vi "Untitled 1.vi"() -> ()   [LabVIEW 2016]
uses:
  PC/llb/granula_llb.lvlib
panel:
  out "текущее время":string
  out "ВЫХОД 2":bool
  in  "x140":i32
  in  "x200":i32
  in  "x240":i32
  in  "y60":i32
  in  "y120":i32
  in  "x100":i32
  in  "x300":i32
  in  "x340":i32
  in  "x400":i32
  in  "Запись отчета":bool
  in  "V7045_I_ist":dbl
  out "U_ist":string caption="Voltage (V)"
  in  "V7045_U_ist":dbl
  out "Диаметр заг.":string caption="Diameter (mm)"
  in  "out":dbl
  out "Boolean":bool
  in  "PV_зазор":dbl
  in  "задание тока А":string caption="Задание, А"
  in  "Скорость ПП 2":string caption="Plasmatron speed (mm/min)"
  in  "Скорость ПП":string caption="Longitudial speed (mm/min)"
  out "Полож плазм кон":bool caption="Конец"
  out "Полож плазм сер":bool caption="Пром."
  out "Полож заг сер":bool
  out "Полож заг нач":bool caption="НАЧАЛО"
  out "Полож заг кон":bool
  out "Полож плазм  нач":bool caption="Начало"
  out "PE2 5":string caption="Вакуум в камере\nPT2 (torr)"
  out "PE1 4":string caption="Вакуум в камере\nPT2 (torr)"
  out "PE3 5":string caption="Вакуум в камере\nPT2 (torr)"
  in  "PE1 3":dbl
  in  "PE2 4":dbl
  in  "PE3 4":dbl
  out "ИНдикатор положения полки":string
  out "P plasmatron (bar)":string
  out "P camera (bar)":string
  out "Air 2":bool
  out "Water-1 2":bool
  out "Water-2 2":bool
  out "Air 4":bool
  out "PT 8":string caption="Вакуум в камере\nPT2 (torr)"
  out "PT 7":string caption="Вакуум в камере\nPT2 (torr)"
  out "PT 6":string caption="Вакуум в камере\nPT2 (torr)"
  in  "PT1 2":dbl
  in  "PT2 2":dbl
  in  "PT3 3":dbl
  out "PT 5":string caption="Вакуум в камере\nPT2 (torr)"
  in  "PT3 2":dbl
  out "X100":bool[](array[boolean])
  out "X140":bool[](array[boolean])
  out "X200":bool[](array[boolean])
  out "X240":bool[](array[boolean])
  out "X300":bool[](array[boolean])
  out "X340":bool[](array[boolean])
  out "X400":bool[](array[boolean])
  out "Y60":bool[](array[boolean])
  out "Y120":bool[](array[boolean])
  in  "Ошибка":i16
  in  "Т1":dbl
  in  "Т2":dbl
  in  "Т3":dbl
  in  "Т4":dbl
  in  "Т5":dbl
  out "V вращ. бараб":string caption="Rotation frequency (r/min)"
  in  "V барабаны":dbl
  out "V заготовки":string
  out "V задания":string caption="Rotation speed (r/min)"
  in  "V барабаны задание":dbl
  in  "Скорость пп":i16
  in  "ЗАДАНИЕ ТОКА":i16
  in  "откачка стоп индик 3":bool
  out "ПОДШ. 1.1":string caption="T1 (C°)"
  out "ПОДШ. 1.2":string caption="T2 (C°)"
  out "ПОДШ. 2.1":string caption="T3 (C°)"
  out "ПОДШ. 2.2":string caption="T4 (C°)"
  out "ТЕМП РОЛИК":string caption="T roller (C°)"
  out "ТЕМП КАМЕРА":string caption="T gas (C°)"
  in  "Т6":dbl
  in  "Скорость пп 2":i16
  out "V барабаны 2":dbl
  out "voto plasmatron":string caption="MOTO\nPLASMATRON"
  in  "M_PLasmatron":dbl
  out "VOLTAGE":dbl(graph)
  out "CURRENT":dbl(graph)
  out "LONGITUDINAL FEED":dbl(graph)
  out "PV":dbl(graph)
  out "PULLEYS":dbl(graph)
  out "max Speed":string caption="Max speed (r/min)"
  in  "Position (mm)":dbl(slide) scale=0.0..820.0
  out "String":string
  out "ролик_прижат":bool caption="Down"
  out "ролик_отжат":bool caption="Up"
  out "УГ_открыт":bool caption="Open"
  out "УГ_закрыт":bool caption="Close"
  in  "Выход":bool
  in  "Tab Control":enum32{"VACUUM"}(tab)
  out "PT3":u16(ring)
  out "PT 3":string caption="Вакуум в камере\nPT2 (torr)"
  out "PA":string
  out "PD1":u16(ring)
  out "VP8":u16(ring)
  out "PA1":string
  out "PD2":u16(ring)
  in  "forvacuum":bool
  in  "forvakuum led":bool
  in  "Slide":dbl(slide) scale=0.0..99.0
  out "NL 2":u16(ring)
  out "VP9":u16(ring)
  in  "ND HEAT BUT":bool
  in  "ND HEAT LED":bool
  in  "откачка стоп 2":bool
  in  "откачка стоп индик 2":bool
  out "Water-2":bool
  out "Water-1":bool
  out "Air":bool
  in  "откачка стоп":bool
  in  "откачка стоп индик":bool
  out "EV1":u16(ring)
  out "EV2":u16(ring)
  out "EV3.3":u16(ring)
  out "EV3.2":u16(ring)
  out "PE2":u16(ring)
  out "PE2":string caption="Вакуум в камере\nPT2 (torr)"
  out "CO1":u16(ring)
  out "CO2":u16(ring)
  out "EV3.1":u16(ring)
  out "CO3":u16(ring)
  out "P1":u16(ring)
  out "PE1":u16(ring)
  out "PE1":string caption="Вакуум в камере\nPT2 (torr)"
  out "PE3":u16(ring)
  out "PE3":string caption="Вакуум в камере\nPT2 (torr)"
  out "VP1":u16(ring)
  out "VP2":u16(ring)
  out "PT2":u16(ring)
  out "PT 2":string caption="Вакуум в камере\nPT2 (torr)"
  out "VP3":u16(ring)
  out "VP5":u16(ring)
  out "PT1":u16(ring)
  out "PT 1":string caption="Вакуум в камере\nPT2 (torr)"
  out "NZ":u16(ring)
  out "NB":u16(ring)
  out "NL":u16(ring)
  out "VP7":u16(ring)
  in  "mac 4":bool
  in  "напустить аргон":bool
  in  "откачать рабочий вакуум":bool
  in  "mac 2":bool
  # "VF1"
  # "Ar,He"
  # "PC1"
  # "PC2"
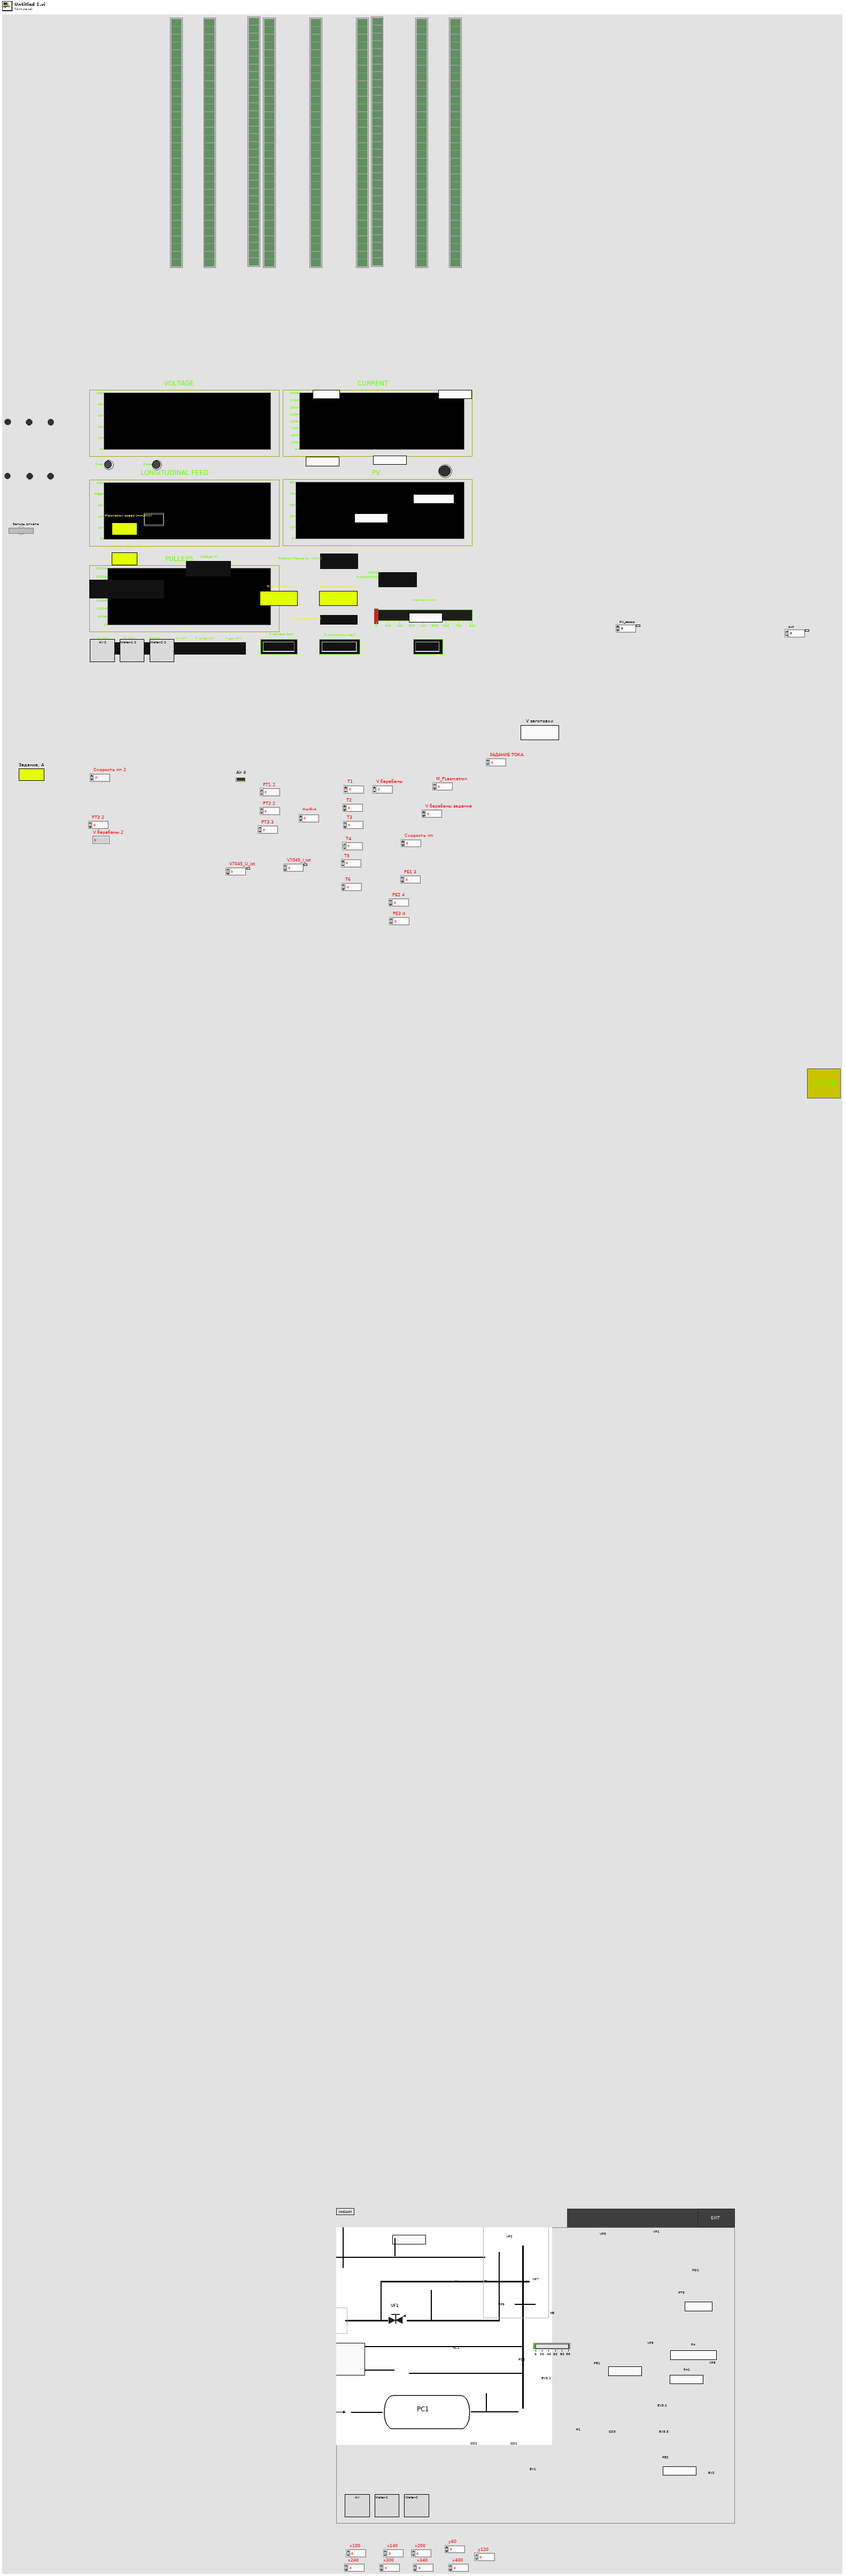
[diagram p1: front panel]
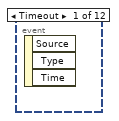
[diagram p2: hidden frame]
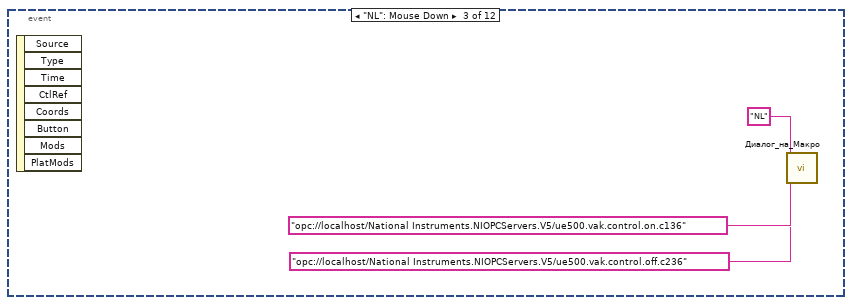
[diagram p3: hidden frame]
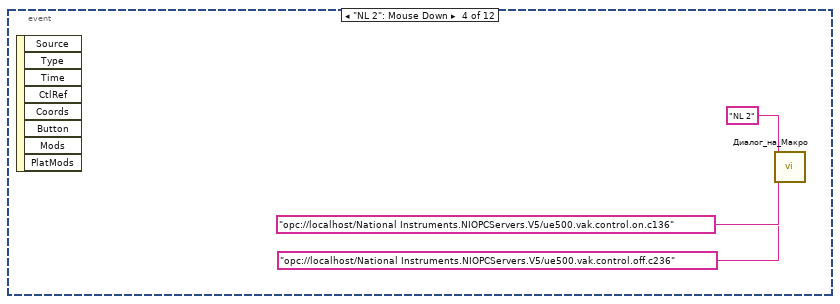
[diagram p4: hidden frame]
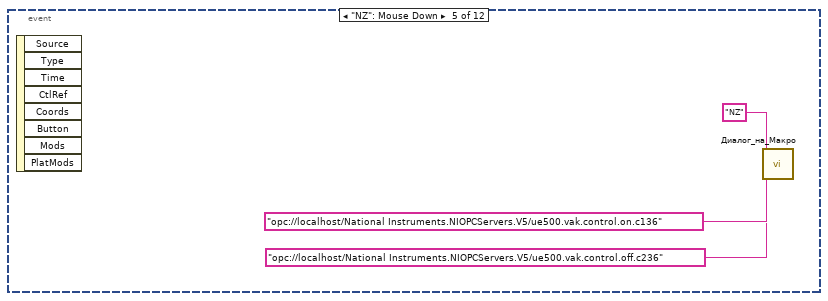
[diagram p5: hidden frame]
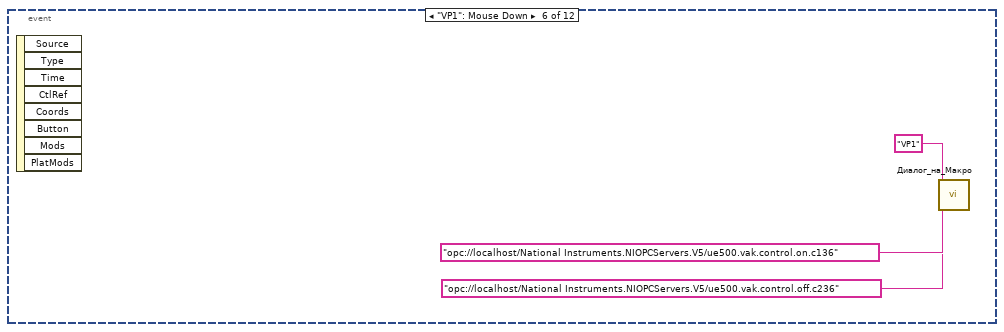
[diagram p6: hidden frame]
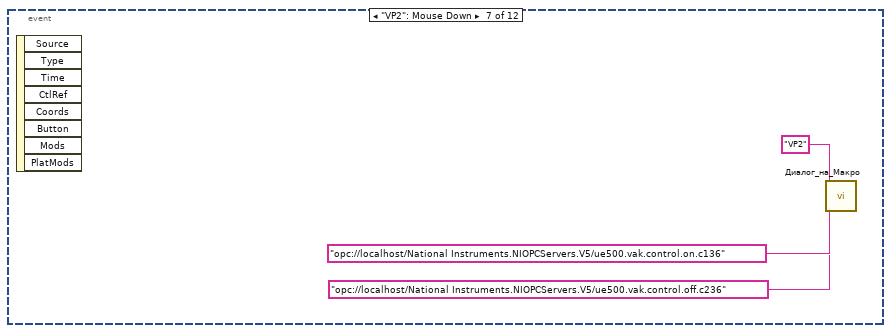
[diagram p7: hidden frame]
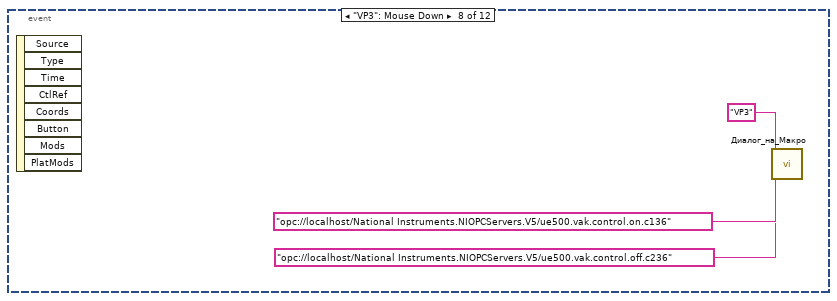
[diagram p8: hidden frame]
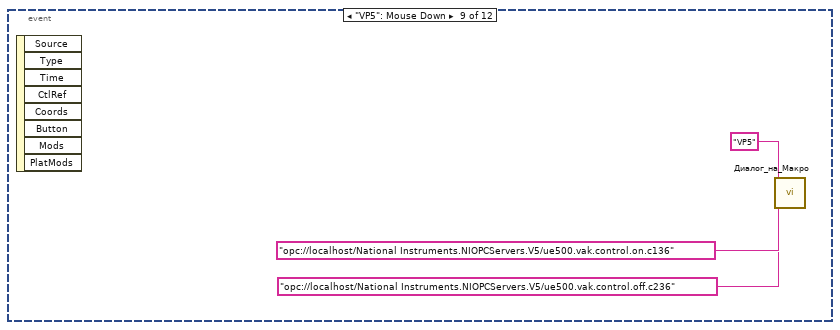
[diagram p9: hidden frame]
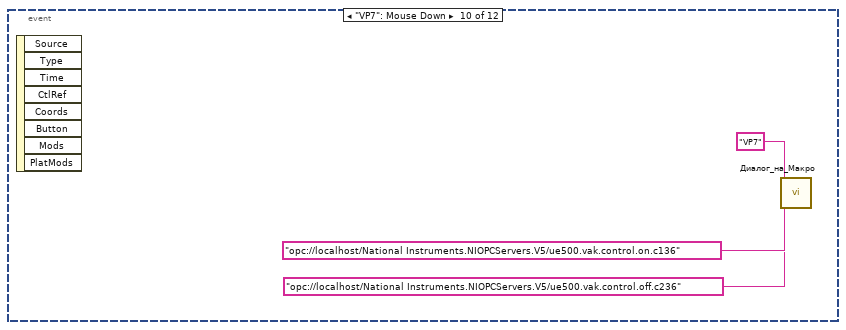
[diagram p10: hidden frame]
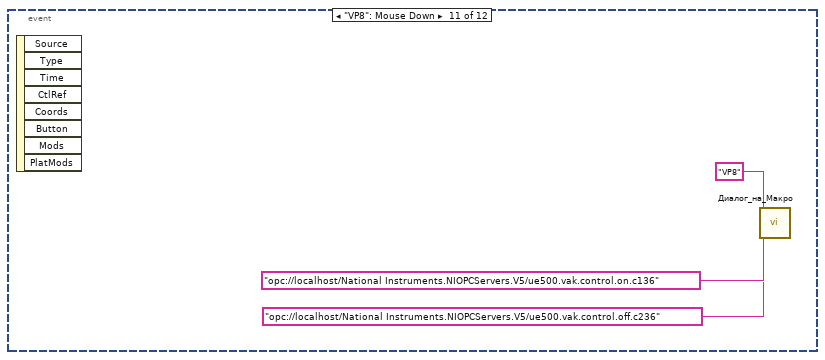
[diagram p11: hidden frame]
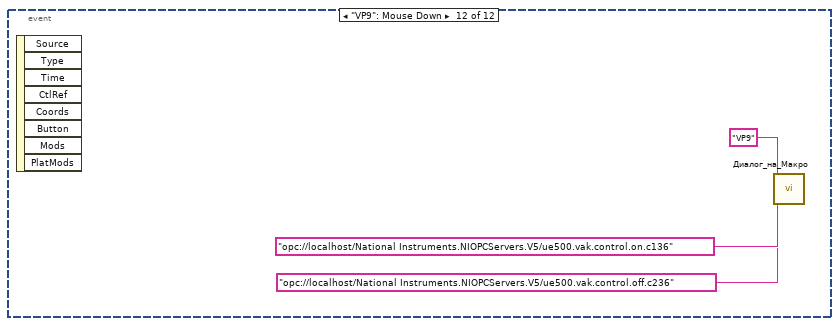
[diagram p12: hidden frame]
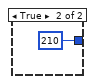
[diagram p13: hidden frame]
diagram:
  n1 = flat-sequence {
    frame #0 {
      n2 = while {
        stop <- FALSE stop-if-true
        w110 = i16 1 ("precision (6)")
        # "Вакуумная"
        n3 = local read "Y120"() -> (w228:bool[])
        n4 = local read "X200"() -> (w290:bool[])
        n5 = local read "X240"() -> (w274:bool[])
        n6 = local read "X100"() -> (w126:bool[])
        n7 = local read "X300"() -> (w249:bool[])
        n8 = local read "X340"() -> (w235:bool[])
        n9 = local read "X140"() -> (w309:bool[])
        n10 = local read "X400"() -> (w176:bool[])
        n11 = local read "Y60"() -> (w229:bool[])
        n12 = local read "out"() -> (→"LONGITUDINAL FEED":dbl)
        n13 = Get Date/Time In Seconds() -> (seconds since 1Jan1904=w183:timestamp)
        n14 = Wait Until Next ms Multiple(millisecond multiple=u32 500) -> ()  [unwired: 1 out]
        n15 = local read "V7045_U_ist"() -> (→"VOLTAGE":dbl)
        n16 = local read "V7045_I_ist"() -> (→"CURRENT":dbl)
        n17 = local read "PV_зазор"() -> (→"PV":dbl)
        n18 = local read "X140"() -> (w153:bool[])
        n19 = call "Метакон.vi"("Vak_in"="PT2 2") -> ("Vak_out_txt"=→"PT 7":string)  [unwired: 9 in, 1 out]
        n20 = call "Метакон.vi"("Vak_in"="PT3 3") -> ("Vak_out_txt"=→"PT 6":string)  [unwired: 9 in, 1 out]
        n21 = call "Метакон.vi"("Vak_in"="PT1 2") -> ("Vak_out_txt"=→"PT 8":string)  [unwired: 9 in, 1 out]
        n22 = Format Date/Time String(seconds (now)=w183) -> (date/time string=→"текущее время":string)  [unwired: 2 in]
        n23 = Number To Fractional String(number="Т1", precision (6)=w110) -> (F-format string=→"ПОДШ. 1.1":string)  [unwired: 2 in]
        n24 = Number To Fractional String(number="Т2", precision (6)=w110) -> (F-format string=→"ПОДШ. 1.2":string)  [unwired: 2 in]
        n25 = Number To Fractional String(number="Т3", precision (6)=w110) -> (F-format string=→"ПОДШ. 2.1":string)  [unwired: 2 in]
        n26 = Number To Fractional String(number="Т4", precision (6)=w110) -> (F-format string=→"ПОДШ. 2.2":string)  [unwired: 2 in]
        n27 = Number To Fractional String(number="Т5", precision (6)=w110) -> (F-format string=→"ТЕМП РОЛИК":string)  [unwired: 2 in]
        n28 = Number To Fractional String(number="Т6", precision (6)=w110) -> (F-format string=→"ТЕМП КАМЕРА":string)  [unwired: 2 in]
        n29 = call "presure PA.vi"("Volte"="PT3 2") -> ("presure String 2"=→"PT 5":string)  [unwired: 7 in, 3 out]
        n30 = Number To Boolean Array(number="x340") -> (Boolean array=→"X340":bool[])
        n31 = Number To Boolean Array(number="x200") -> (Boolean array=→"X200":bool[])
        n32 = Number To Boolean Array(number="x400") -> (Boolean array=→"X400":bool[])
        n33 = Number To Boolean Array(number="y120") -> (Boolean array=→"Y120":bool[])
        n34 = Number To Boolean Array(number="x140") -> (Boolean array=→"X140":bool[])
        n35 = Number To Boolean Array(number="x300") -> (Boolean array=→"X300":bool[])
        n36 = Number To Boolean Array(number="x240") -> (Boolean array=→"X240":bool[])
        n37 = Number To Boolean Array(number="x100") -> (Boolean array=→"X100":bool[])
        n38 = Number To Boolean Array(number="y60") -> (Boolean array=→"Y60":bool[])
        n39 = local read "V вращ. бараб"() -> (w201:string)
        n40 = local read "V барабаны 2"() -> (→"PULLEYS":dbl)
        n41 = Index Array(array=w235, index #1=2, index #2=5) -> ()  [unwired: 2 out]
        n42 = Number To Fractional String(number="PE3 4", precision (6)=i16 2) -> (F-format string=→"PE3 5" →"P camera (bar)":string)  [unwired: 2 in]
        n43 = Number To Fractional String(number="PE1 3", precision (6)=i16 2) -> (F-format string=→"PE1 4" →"P plasmatron (bar)":string)  [unwired: 2 in]
        n44 = Number To Fractional String(number="PE2 4", precision (6)=i16 1) -> (F-format string=→"PE2 5":string)  [unwired: 2 in]
        n45 = local read "Диаметр заг."() -> (w118:string)
        n46 = Index Array(array=w229, index #1=10, index #2=11, index #3=12) -> (element #1=w223:bool, element #2=w222:bool, element #3=w221:bool)
        n47 = Index Array(array=w176, index #1=27, index #2=29, index #3=30) -> (element #1=w180:bool, element #2=w181:bool, element #3=w182:bool)
        n48 = Index Array(array=w228, index #1=23, index #2=24, index #3=25, index #4=26) -> (element #1=w220:bool, element #2=w219:bool, element #3=w218:bool, element #4=w217:bool)
        n49 = Index Array(array=w309, index #1=16, index #2=18, index #3=19, index #4=20, index #5=21, index #6=24, index #7=25, index #8=28, index #9=29) -> (element #6=→"ролик_прижат":bool, element #7=→"ролик_отжат":bool, element #8=→"УГ_открыт":bool, element #9=→"УГ_закрыт":bool)  [unwired: 5 out]
        n50 = local read "U_ist"() -> (w196:string)
        n51 = To Long Integer(number="Скорость пп 2") -> (32bit integer=w115:i32)
        n52 = To Long Integer(number="Скорость пп") -> (32bit integer=w91:i32)
        n53 = Index Array(array=w290, index #1=1, index #2=6, index #3=7, index #4=27, index #5=14, index #6=13, index #7=21, index #8=22, index #9=23, index #10=24, index #11=25, index #12=19) -> ()  [unwired: 12 out]
        n54 = Index Array(array=w126, index #1=2, index #2=5, index #3=8, index #4=12, index #5=11, index #6=17, index #7=16, index #8=21, index #9=20, index #10=25, index #11=24, index #12=29, index #13=28) -> (element #1=w128:bool, element #2=w130:bool, element #3=w131:bool, element #4=w133:bool, element #5=w134:bool, element #6=w137:bool, element #7=w138:bool, element #8=w145:bool, element #9=w146:bool, element #10=w147:bool, element #11=w148:bool, element #12=w151:bool, element #13=w152:bool)
        n55 = Number To Fractional String(number="M_PLasmatron", precision (6)=i16 1) -> (F-format string=→"voto plasmatron":string)  [unwired: 2 in]
        n56 = Index Array(array=w274, index #1=16, index #2=17, index #3=18, index #4=19, index #5=20, index #6=9, index #7=12, index #8=13, index #9=16, index #10=17, index #11=18, index #12=19, index #13=21, index #14=22, index #15=23, index #16=27, index #17=28, index #18=29) -> (element #1=→"Air 2":bool, element #2=→"Air 4":bool, element #3=→"Water-1 2":bool, element #4=→"Water-2 2":bool)  [unwired: 14 out]
        n57 = Index Array(array=w249, index #1=0, index #2=1, index #3=8, index #4=9, index #5=12, index #6=13, index #7=20, index #8=21, index #9=22, index #10=23, index #11=24, index #12=25, index #13=26, index #14=27, index #15=28, index #16=29, index #17=30, index #18=31) -> (element #7=w248:bool, element #8=w247:bool, element #9=w246:bool, element #10=w245:bool, element #11=w244:bool, element #12=w243:bool, element #13=w242:bool, element #14=w241:bool, element #15=w240:bool, element #16=w239:bool, element #17=w238:bool)  [unwired: 7 out]
        n58 = Index Array(array=w153, index #1=4, index #2=5, index #3=6, index #4=9, index #5=8, index #6=11, index #7=10) -> (element #1=w161:bool, element #2=w162:bool, element #3=w163:bool, element #4=w164:bool, element #5=w165:bool, element #6=w173:bool, element #7=w172:bool)
        n59 = call "Индекс картинки.vi"("off"=w182, "on"=w181) -> ("index_image"=→"VP9":u16)  [unwired: 9 in]
        n60 = Decimal String To Number(string=w196) -> (number=w195:i32)  [unwired: 2 in, 1 out]
        n61 = Decimal String To Number(string=w201) -> (number=w200:i32)  [unwired: 2 in, 1 out]
        n62 = Boolean To (0,1)(Boolean=w223) -> (0, 1=→"EV1":i16)
        n63 = Boolean To (0,1)(Boolean=w222) -> (0, 1=→"EV2":i16)
        n64 = Boolean To (0,1)(Boolean=w220) -> (0, 1=→"CO1":i16)
        n65 = Boolean To (0,1)(Boolean=w219) -> (0, 1=→"CO2":i16)
        n66 = Boolean To (0,1)(Boolean=w218) -> (0, 1=→"CO3":i16)
        n67 = Boolean To (0,1)(Boolean=w217) -> (0, 1=→"P1":i16)
        n68 = Decimal String To Number(string=w118) -> (number=w81:i32)  [unwired: 2 in, 1 out]
        n69 = Boolean To (0,1)(Boolean=w180) -> (0, 1=→"NL 2":i16)
        n70 = Number To Decimal String(number=w115) -> (decimal integer string=w117:string)  [unwired: 1 in]
        n71 = Number To Decimal String(number=w91) -> (decimal integer string=w92:string)  [unwired: 1 in]
        n72 = Boolean To (0,1)(Boolean=w221) -> (0, 1=→"EV3.2" →"EV3.3" →"EV3.1":i16)
        n73 = Number To Fractional String(number="V барабаны задание", precision (6)=i16 0) -> (F-format string=→"V задания":string)  [unwired: 2 in]
        n74 = Multiply(x="ЗАДАНИЕ ТОКА", y=1.638) -> (x*y=w95:dbl)
        n75 = call "Индекс картинки.vi"("off"=w134, "on"=w133) -> ("index_image"=→"VP1":u16)  [unwired: 9 in]
        n76 = call "Индекс картинки.vi"("off"=w138, "on"=w137) -> ("index_image"=→"VP2":u16)  [unwired: 9 in]
        n77 = call "Индекс картинки.vi"("off"=w146, "on"=w145) -> ("index_image"=→"VP3":u16)  [unwired: 9 in]
        n78 = call "Индекс картинки.vi"("off"=w148, "on"=w147) -> ("index_image"=→"VP7":u16)  [unwired: 9 in]
        n79 = call "Индекс картинки.vi"("off"=w152, "on"=w151) -> ("index_image"=→"VP5":u16)  [unwired: 9 in]
        n80 = call "Индекс картинки.vi"("off"=w165, "on"=w164) -> ("index_image"=→"PD1":u16)  [unwired: 9 in]
        n81 = call "Индекс картинки.vi"("off"=w173, "on"=w172) -> ("index_image"=→"PD2":u16)  [unwired: 9 in]
        n82 = local write "Скорость ПП 2"(w117) -> ()
        n83 = local write "Скорость ПП"(w92) -> ()
        n84 = Boolean To (0,1)(Boolean=w128) -> (0, 1=→"NL":i16)
        n85 = Boolean To (0,1)(Boolean=w131) -> (0, 1=→"NB":i16)
        n86 = Boolean To (0,1)(Boolean=w130) -> (0, 1=→"NZ":i16)
        n87 = Boolean To (0,1)(Boolean=w163) -> (0, 1=→"PT3":i16)
        n88 = Boolean To (0,1)(Boolean=w161) -> (0, 1=→"PT1":i16)
        n89 = Boolean To (0,1)(Boolean=w162) -> (0, 1=→"PT2":i16)
        n90 = Equal?(x=w81, y=0) -> (x = y?=w84:bool)
        n91 = Greater Or Equal?(x=w195, y=20) -> (x >= y?=w193:bool)
        n92 = Greater Or Equal?(x=w200, y=500) -> (x >= y?=w198:bool)
        n93 = Build Array(w248, w247, w246, w245, w244, w243, w242, w241, w240, w239, w238) -> (w209:bool[])
        n94 = And(x=w193, y=w198) -> (x .and. y?=w197:bool)
        n95 = To Long Integer(number=w95) -> (32bit integer=w96:i32)
        n96 = local write "Запись отчета"(w197) -> ()
        n97 = call "1.1 индикар полки.vi"("appended array"=w209) -> ("текущее положение"=→"ИНдикатор положения полки":string)  [unwired: 10 in]
        n98 = Number To Decimal String(number=w96) -> (decimal integer string=w97:string)  [unwired: 1 in]
        n99 = case shown="False" w84 {
          tunnel: w81 -> [w310 _]
          tunnel: [w310 210] -> w80
          frame False {
          }
          frame True {
          }
        }
        n100 = local write "задание тока А"(w97) -> ()
        n101 = Divide(x=210.0, y=w80) -> (x/y=w78:dbl)
        n102 = Number To Decimal String(number="Position (mm)") -> (decimal integer string=→"String":string)  [unwired: 1 in]
        n103 = Multiply(x=9180, y=w78) -> (x*y=w76:dbl)
        n104 = Number To Fractional String(number=w76, precision (6)=i16 0) -> (F-format string=→"max Speed":string)  [unwired: 2 in]
        n105 = Multiply(x="V барабаны", y=w78) -> (x*y=w122:dbl)
        n106 = To Long Integer(number=w122) -> (32bit integer=w83:i32)
        "V барабаны 2" <- w83
        n107 = Number To Fractional String(number=w83, precision (6)=i16 0) -> (F-format string=→"V вращ. бараб":string)  [unwired: 2 in]
      }
      n108 = while {
        stop <- FALSE stop-if-true
        n109 = event shown="[0] \"Выход\": Value Change" {
          selector: _ -> [_]
          dyn-events: _ -> [_]
          timeout: _ -> [_]
          event "Выход": Value Change {
            n110 = event-data() -> ()  [unwired: 1 in, 6 out]
            n111 = Stop(stop? (T)="Выход") -> ()
          }
        }
        n112 = Wait Until Next ms Multiple(millisecond multiple=u32 500) -> ()  [unwired: 1 out]
      }
      n113 = while {
        stop <- w3 stop-if-true
        n114 = event shown="[1] \"NB\": Mouse Down" {
          selector: _ -> [_ _ _ _ _ _ _ _ _ _ _ _]
          dyn-events: _ -> [_ _ _ _ _ _ _ _ _ _ _ _]
          timeout: 100 -> [_ _ _ _ _ _ _ _ _ _ _ _]
          event Timeout {
            n115 = event-data() -> ()  [unwired: 1 in, 3 out]
          }
          event "NB": Mouse Down {
            n116 = event-data() -> ()  [unwired: 1 in, 8 out]
            n117 = call "Диалог_на_Макро.vi"("АДРЕС ДЛЯ ЗАПИСИ ЗАКР\\ОТКЛ"="opc://localhost/National Instruments.NIOPCServers.V5/ue500.vak.control.off.c236" ("АДРЕС ДЛЯ ЗАПИСИ ЗАКР\\ОТКЛ"), "АДРЕС ДЛЯ ЗАПИСИ ОТКР\\ВКД"="opc://localhost/National Instruments.NIOPCServers.V5/ue500.vak.control.on.c136" ("АДРЕС ДЛЯ ЗАПИСИ ОТКР\\ВКД"), "ОПИСАНИЕ"="NB") -> ()  [unwired: 9 in]
          }
          event "NL": Mouse Down {
            n118 = event-data() -> ()  [unwired: 1 in, 8 out]
            n119 = call "Диалог_на_Макро.vi"("АДРЕС ДЛЯ ЗАПИСИ ЗАКР\\ОТКЛ"="opc://localhost/National Instruments.NIOPCServers.V5/ue500.vak.control.off.c236" ("АДРЕС ДЛЯ ЗАПИСИ ЗАКР\\ОТКЛ"), "АДРЕС ДЛЯ ЗАПИСИ ОТКР\\ВКД"="opc://localhost/National Instruments.NIOPCServers.V5/ue500.vak.control.on.c136" ("АДРЕС ДЛЯ ЗАПИСИ ОТКР\\ВКД"), "ОПИСАНИЕ"="NL") -> ()  [unwired: 9 in]
          }
          event "NL 2": Mouse Down {
            n120 = event-data() -> ()  [unwired: 1 in, 8 out]
            n121 = call "Диалог_на_Макро.vi"("АДРЕС ДЛЯ ЗАПИСИ ЗАКР\\ОТКЛ"="opc://localhost/National Instruments.NIOPCServers.V5/ue500.vak.control.off.c236" ("АДРЕС ДЛЯ ЗАПИСИ ЗАКР\\ОТКЛ"), "АДРЕС ДЛЯ ЗАПИСИ ОТКР\\ВКД"="opc://localhost/National Instruments.NIOPCServers.V5/ue500.vak.control.on.c136" ("АДРЕС ДЛЯ ЗАПИСИ ОТКР\\ВКД"), "ОПИСАНИЕ"="NL 2") -> ()  [unwired: 9 in]
          }
          event "NZ": Mouse Down {
            n122 = event-data() -> ()  [unwired: 1 in, 8 out]
            n123 = call "Диалог_на_Макро.vi"("АДРЕС ДЛЯ ЗАПИСИ ЗАКР\\ОТКЛ"="opc://localhost/National Instruments.NIOPCServers.V5/ue500.vak.control.off.c236" ("АДРЕС ДЛЯ ЗАПИСИ ЗАКР\\ОТКЛ"), "АДРЕС ДЛЯ ЗАПИСИ ОТКР\\ВКД"="opc://localhost/National Instruments.NIOPCServers.V5/ue500.vak.control.on.c136" ("АДРЕС ДЛЯ ЗАПИСИ ОТКР\\ВКД"), "ОПИСАНИЕ"="NZ") -> ()  [unwired: 9 in]
          }
          event "VP1": Mouse Down {
            n124 = event-data() -> ()  [unwired: 1 in, 8 out]
            n125 = call "Диалог_на_Макро.vi"("АДРЕС ДЛЯ ЗАПИСИ ЗАКР\\ОТКЛ"="opc://localhost/National Instruments.NIOPCServers.V5/ue500.vak.control.off.c236" ("АДРЕС ДЛЯ ЗАПИСИ ЗАКР\\ОТКЛ"), "АДРЕС ДЛЯ ЗАПИСИ ОТКР\\ВКД"="opc://localhost/National Instruments.NIOPCServers.V5/ue500.vak.control.on.c136" ("АДРЕС ДЛЯ ЗАПИСИ ОТКР\\ВКД"), "ОПИСАНИЕ"="VP1") -> ()  [unwired: 9 in]
          }
          event "VP2": Mouse Down {
            n126 = event-data() -> ()  [unwired: 1 in, 8 out]
            n127 = call "Диалог_на_Макро.vi"("АДРЕС ДЛЯ ЗАПИСИ ЗАКР\\ОТКЛ"="opc://localhost/National Instruments.NIOPCServers.V5/ue500.vak.control.off.c236" ("АДРЕС ДЛЯ ЗАПИСИ ЗАКР\\ОТКЛ"), "АДРЕС ДЛЯ ЗАПИСИ ОТКР\\ВКД"="opc://localhost/National Instruments.NIOPCServers.V5/ue500.vak.control.on.c136" ("АДРЕС ДЛЯ ЗАПИСИ ОТКР\\ВКД"), "ОПИСАНИЕ"="VP2") -> ()  [unwired: 9 in]
          }
          event "VP3": Mouse Down {
            n128 = event-data() -> ()  [unwired: 1 in, 8 out]
            n129 = call "Диалог_на_Макро.vi"("АДРЕС ДЛЯ ЗАПИСИ ЗАКР\\ОТКЛ"="opc://localhost/National Instruments.NIOPCServers.V5/ue500.vak.control.off.c236" ("АДРЕС ДЛЯ ЗАПИСИ ЗАКР\\ОТКЛ"), "АДРЕС ДЛЯ ЗАПИСИ ОТКР\\ВКД"="opc://localhost/National Instruments.NIOPCServers.V5/ue500.vak.control.on.c136" ("АДРЕС ДЛЯ ЗАПИСИ ОТКР\\ВКД"), "ОПИСАНИЕ"="VP3") -> ()  [unwired: 9 in]
          }
          event "VP5": Mouse Down {
            n130 = event-data() -> ()  [unwired: 1 in, 8 out]
            n131 = call "Диалог_на_Макро.vi"("АДРЕС ДЛЯ ЗАПИСИ ЗАКР\\ОТКЛ"="opc://localhost/National Instruments.NIOPCServers.V5/ue500.vak.control.off.c236" ("АДРЕС ДЛЯ ЗАПИСИ ЗАКР\\ОТКЛ"), "АДРЕС ДЛЯ ЗАПИСИ ОТКР\\ВКД"="opc://localhost/National Instruments.NIOPCServers.V5/ue500.vak.control.on.c136" ("АДРЕС ДЛЯ ЗАПИСИ ОТКР\\ВКД"), "ОПИСАНИЕ"="VP5") -> ()  [unwired: 9 in]
          }
          event "VP7": Mouse Down {
            n132 = event-data() -> ()  [unwired: 1 in, 8 out]
            n133 = call "Диалог_на_Макро.vi"("АДРЕС ДЛЯ ЗАПИСИ ЗАКР\\ОТКЛ"="opc://localhost/National Instruments.NIOPCServers.V5/ue500.vak.control.off.c236" ("АДРЕС ДЛЯ ЗАПИСИ ЗАКР\\ОТКЛ"), "АДРЕС ДЛЯ ЗАПИСИ ОТКР\\ВКД"="opc://localhost/National Instruments.NIOPCServers.V5/ue500.vak.control.on.c136" ("АДРЕС ДЛЯ ЗАПИСИ ОТКР\\ВКД"), "ОПИСАНИЕ"="VP7") -> ()  [unwired: 9 in]
          }
          event "VP8": Mouse Down {
            n134 = event-data() -> ()  [unwired: 1 in, 8 out]
            n135 = call "Диалог_на_Макро.vi"("АДРЕС ДЛЯ ЗАПИСИ ЗАКР\\ОТКЛ"="opc://localhost/National Instruments.NIOPCServers.V5/ue500.vak.control.off.c236" ("АДРЕС ДЛЯ ЗАПИСИ ЗАКР\\ОТКЛ"), "АДРЕС ДЛЯ ЗАПИСИ ОТКР\\ВКД"="opc://localhost/National Instruments.NIOPCServers.V5/ue500.vak.control.on.c136" ("АДРЕС ДЛЯ ЗАПИСИ ОТКР\\ВКД"), "ОПИСАНИЕ"="VP8") -> ()  [unwired: 9 in]
          }
          event "VP9": Mouse Down {
            n136 = event-data() -> ()  [unwired: 1 in, 8 out]
            n137 = call "Диалог_на_Макро.vi"("АДРЕС ДЛЯ ЗАПИСИ ЗАКР\\ОТКЛ"="opc://localhost/National Instruments.NIOPCServers.V5/ue500.vak.control.off.c236" ("АДРЕС ДЛЯ ЗАПИСИ ЗАКР\\ОТКЛ"), "АДРЕС ДЛЯ ЗАПИСИ ОТКР\\ВКД"="opc://localhost/National Instruments.NIOPCServers.V5/ue500.vak.control.on.c136" ("АДРЕС ДЛЯ ЗАПИСИ ОТКР\\ВКД"), "ОПИСАНИЕ"="VP9") -> ()  [unwired: 9 in]
          }
        }
        n138 = Wait Until Next ms Multiple(millisecond multiple=u32 500) -> ()  [unwired: 1 out]
        n139 = local read "ВЫХОД 2"() -> (w3:bool)
      }
    }
  }
